vi "cno_check parameters.vi"(4 "initial parameters":dbl[](array[numeric]), 7 "tuning parameters":T7={"constraint weight"=1.0, "maximum minor iterations"=10}, 8 "error in (no error)":errorcluster, 9 "user defined functions":T2, 10 "limits":T5, 11 "state values":T6) -> (0 "error out":errorcluster, 1 "OB0":dbl[](array[numeric]), 2 "limits out":T5, 3 "state values out":T6, 5 "cno data":T1)   [LabVIEW 2017, in "NI_Gmath.lvlib"]
uses:
  <vilib>/gmath/NI_Gmath.lvlib
  <vilib>/gmath/NumericalOptimization/cno_initial values.ctl
  <vilib>/gmath/NumericalOptimization/cno_bounds.ctl
  <vilib>/gmath/NumericalOptimization/cno_tuning parameters.ctl
  <vilib>/gmath/NumericalOptimization/cno_user defined functions.ctl
  <vilib>/gmath/NumericalOptimization/cno_user objective function ref.ctl
  <vilib>/gmath/NumericalOptimization/objective function data.ctl
  <vilib>/gmath/NumericalOptimization/cno_data.ctl
  <vilib>/Analysis/7linalg.llb/Create Special Real Matrix.vi
  <vilib>/gmath/NumericalOptimization/zeroes_1d.vi
  <vilib>/Analysis/NI_AALPro.lvlib
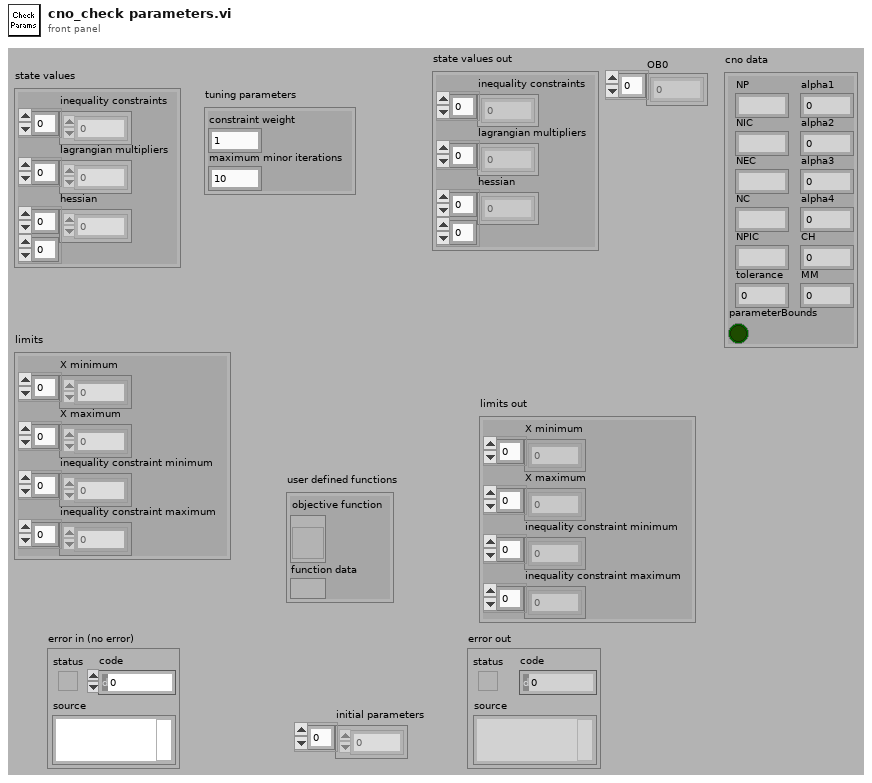
[diagram p1: front panel]
types:
  T1 = typedef "NI_Gmath.lvlib/cno_data.ctl" = cluster{"NP":i32, "NIC":i32, "NEC":i32, "NC":i32, "NPIC":i32, "parameterBounds":bool, "alpha1":dbl, "alpha2":dbl, "alpha3":dbl, "alpha4":dbl, "CH":i32, "MM":i32, "tolerance":dbl}
  T2 = typedef "NI_Gmath.lvlib/cno_user defined functions.ctl" = cluster{"objective function":T3, "function data":T4}
  T3 = typedef "NI_Gmath.lvlib/cno_user objective function ref.ctl" = refnum<vi>
  T4 = typedef "NI_Gmath.lvlib/objective function data.ctl" = variant
  T5 = typedef "NI_Gmath.lvlib/cno_bounds.ctl" = cluster{"X minimum":dbl[], "X maximum":dbl[], "inequality constraint minimum":dbl[], "inequality constraint maximum":dbl[]}
  T6 = typedef "NI_Gmath.lvlib/cno_initial values.ctl" = cluster{"inequality constraints":dbl[], "lagrangian multipliers":dbl[], "hessian":dbl[][]}
  T7 = typedef "NI_Gmath.lvlib/cno_tuning parameters.ctl" = cluster{"constraint weight":dbl, "maximum minor iterations":i32}
  T8 = enum32{"Identity", "Diagonal", "Toepliz", "Vandermonde", "Companion"}
  T9 = typedef "NI_Matrix.lvlib/RealMatrix.ctl" = dbl[][]
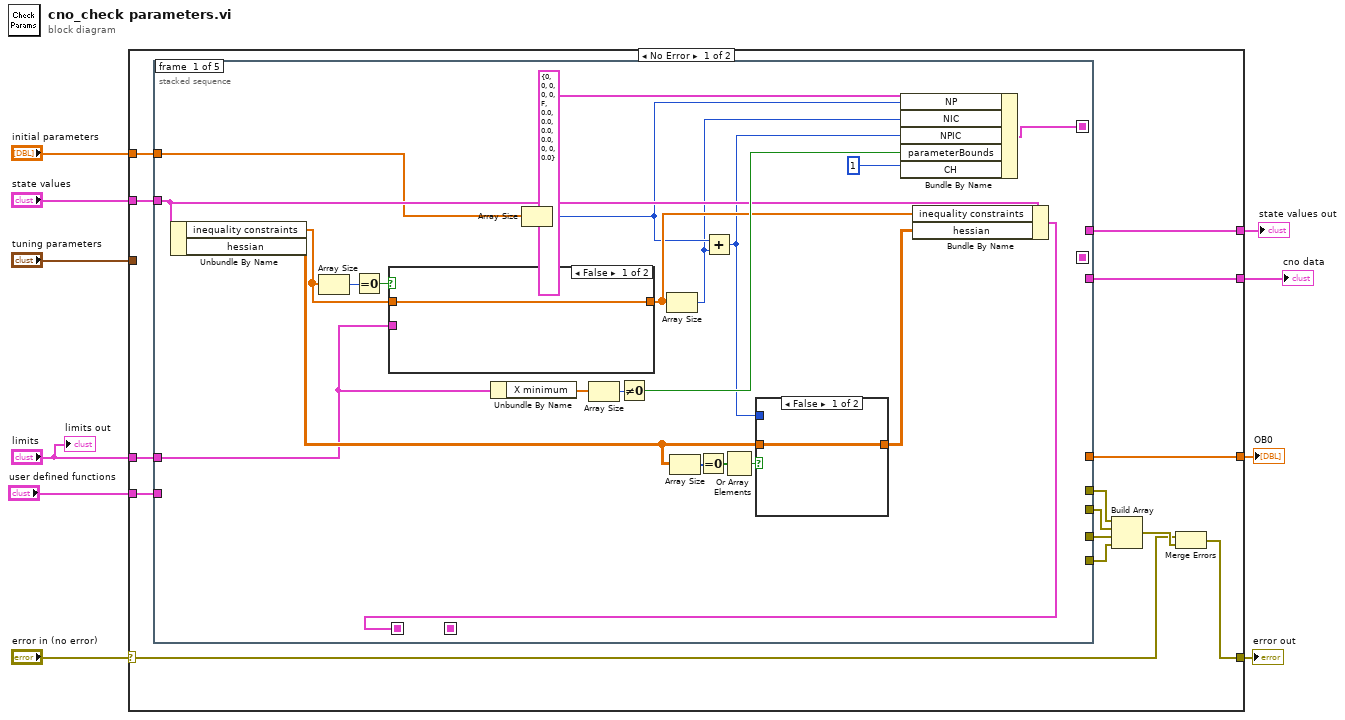
[diagram p0: block diagram]
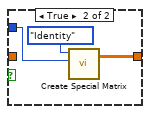
[diagram p2: hidden frame]
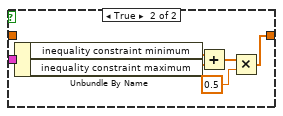
[diagram p3: hidden frame]
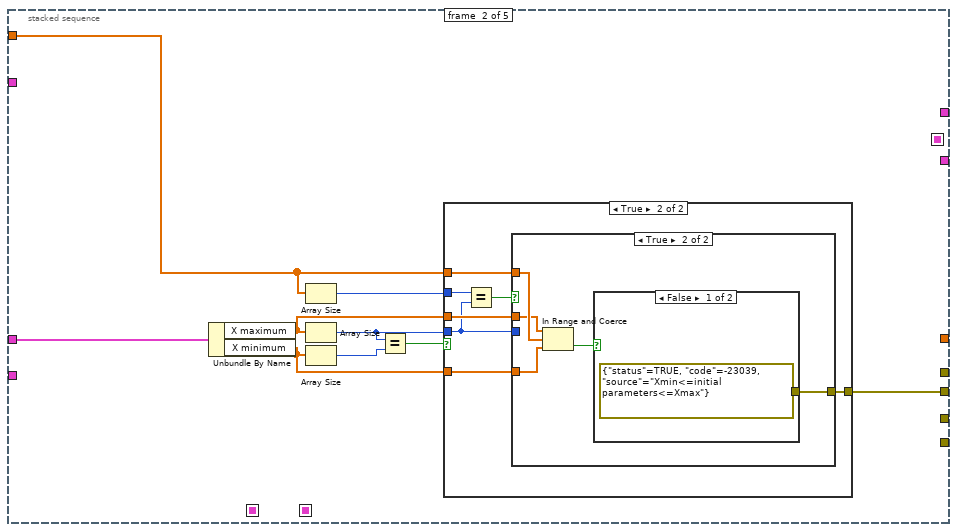
[diagram p4: hidden frame]
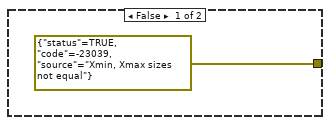
[diagram p5: hidden frame]
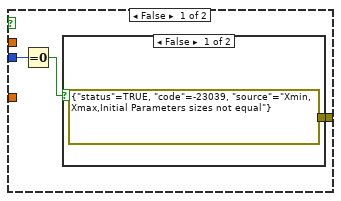
[diagram p6: hidden frame]
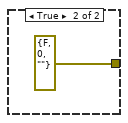
[diagram p8: hidden frame]
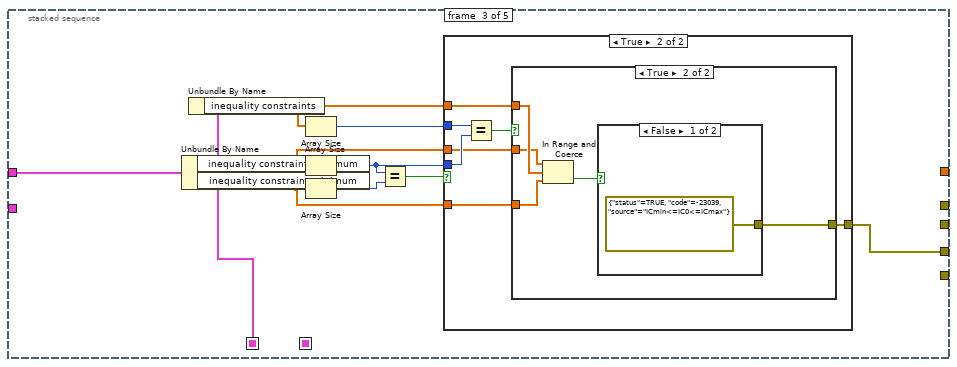
[diagram p9: hidden frame]
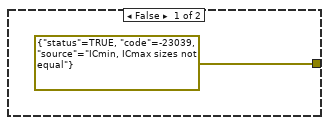
[diagram p10: hidden frame]
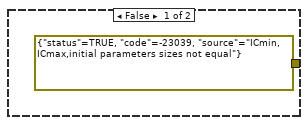
[diagram p11: hidden frame]
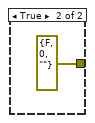
[diagram p12: hidden frame]
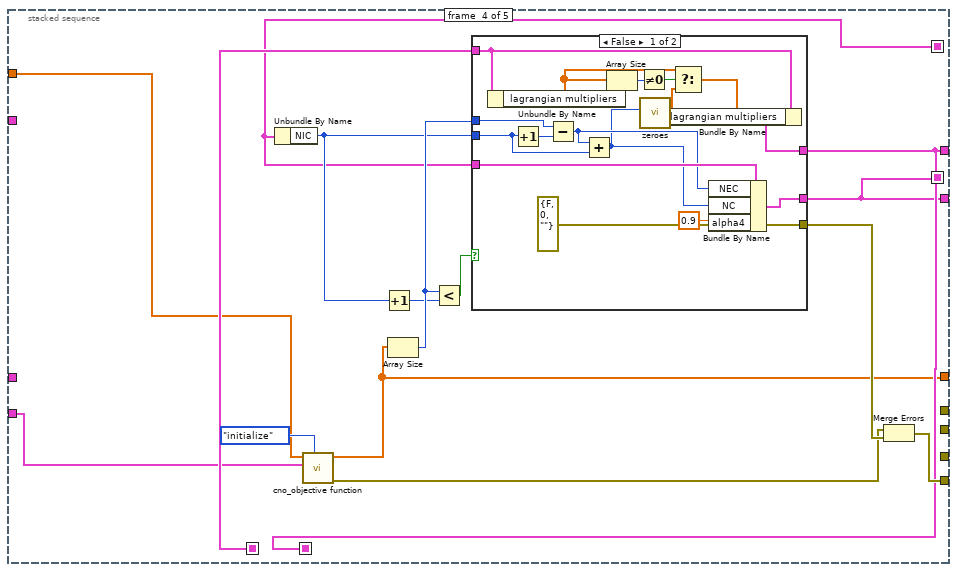
[diagram p13: hidden frame]
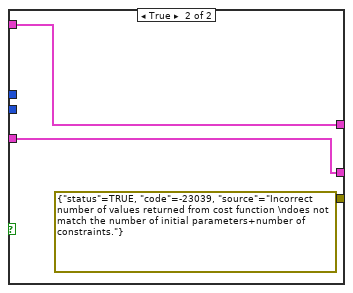
[diagram p14: hidden frame]
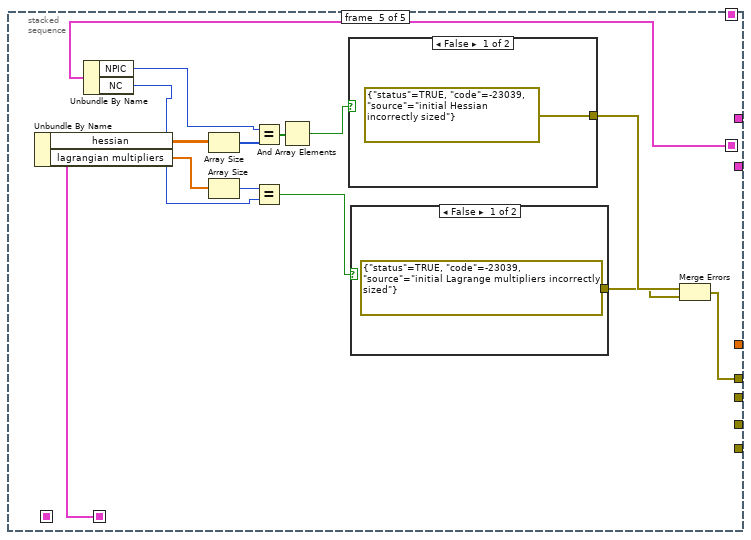
[diagram p15: hidden frame]
diagram:
  n1 = case shown="No Error" "error in (no error)" {
    selector: "error in (no error)" -> [w14 w162]
    tunnel: "tuning parameters" -> [_ _]
    tunnel: "state values" -> [w24 w163]
    tunnel: "limits" -> [w23 _]
    tunnel: [w22 w163] -> w7
    tunnel: [w21 w162] -> w6
    tunnel: [w20 _] -> w4
    tunnel: "user defined functions" -> [w19 _]
    tunnel: [w12 _] -> w2
    tunnel: "initial parameters" -> [w11 _]
    frame No Error {
      n2 = stacked-sequence {
        seq-local: [w40 _ _ _ _] -> [_ _ w86 w123 _]
        seq-local: [_ _ _ w121 _] -> [_ _ _ _ w159]
        seq-local: [w25 _ _ _ _] -> [_ _ _ w113 _]
        seq-local: [_ _ _ w112 _] -> [_ _ _ _ w146]
        tunnel: w24 -> [w45 _ _ _ _]
        tunnel: w23 -> [w31 w66 w95 _ _]
        tunnel: [_ _ _ w121 _] -> w22
        tunnel: [_ w60 _ _ _] -> w18
        tunnel: [_ _ w87 _ _] -> w17
        tunnel: [_ _ _ w115 _] -> w20
        tunnel: w19 -> [_ _ _ w114 _]
        tunnel: [_ _ _ w122 _] -> w16
        tunnel: [_ _ _ _ w149] -> w13
        tunnel: [_ _ _ w112 _] -> w12
        tunnel: w11 -> [w27 w58 _ w116 _]
        frame #0 {
          n3 = Unbundle By Name(w45) -> ("inequality constraints"=w42:dbl[], "hessian"=w35:dbl[][])
          n4 = Array Size(array=w42) -> (size(s)=w44:i32)
          n5 = Equal To 0?(x=w44) -> (x = 0?=w43:bool)
          n6 = case shown="False" w43 {
            tunnel: w31 -> [_ w57]
            tunnel: [w51 w52] -> w41
            tunnel: w42 -> [w51 _]
            frame False {
            }
            frame True {
              n7 = Unbundle By Name(w57) -> ("inequality constraint minimum"=w56:dbl[], "inequality constraint maximum"=w55:dbl[])
              n8 = Add(x=w56, y=w55) -> (x+y=w54:dbl[])
              n9 = Multiply(x=w54, y=0.5) -> (x*y=w52:dbl[])
            }
          }
          n10 = Unbundle By Name(w31) -> ("X minimum"=w30:dbl[])
          n11 = Array Size(array=w27) -> (size(s)=w34:i32)
          n12 = Array Size(array=w30) -> (size(s)=w29:i32)
          n13 = Not Equal To 0?(x=w29) -> (x != 0?=w46:bool)
          n14 = Array Size(array=w41) -> (size(s)=w33:i32)
          n15 = Array Size(array=w35) -> (size(s)=w39:i32[])
          n16 = Equal To 0?(x=w39) -> (x = 0?=w38:bool[])
          n17 = Add(x=w34, y=w33) -> (x+y=w32:i32)
          n18 = Or Array Elements(Boolean array=w38) -> (logical OR=w37:bool)
          n19 = case shown="False" w37 {
            tunnel: [w47 w49] -> w36
            tunnel: w35 -> [w47 _]
            tunnel: w32 -> [_ w48]
            frame False {
            }
            frame True {
              n20 = call-poly <vilib>:"Create Special Matrix.vi"("matrix type"=T8."Identity", "matrix size"=w48) -> ("Special Matrix"=w49:T9)  [unwired: 3 in, 1 out]
            }
          }
          n21 = Bundle By Name(cluster=T1 {"NP"=0, "NIC"=0, "NEC"=0, "NC"=0, "NPIC"=0, "parameterBounds"=FALSE, "alpha1"=0.0, "alpha2"=0.0, "alpha3"=0.0, "alpha4"=0.0, "CH"=0, "MM"=0, "tolerance"=0.0} ("cno data"), "NP"=w34, "NIC"=w33, "NPIC"=w32, "parameterBounds"=w46, "CH"=1) -> (w25:T1)
          n22 = Bundle By Name(cluster=w45, "inequality constraints"=w41, "hessian"=w36) -> (w40:T6)
        }
        frame #1 {
          n23 = Unbundle By Name(w66) -> ("X maximum"=w62:dbl[], "X minimum"=w61:dbl[])
          n24 = Array Size(array=w58) -> (size(s)=w63:i32)
          n25 = Array Size(array=w62) -> (size(s)=w59:i32)
          n26 = Array Size(array=w61) -> (size(s)=w65:i32)
          n27 = Equal?(x=w59, y=w65) -> (x = y?=w64:bool)
          n28 = case shown="True" w64 {
            tunnel: w63 -> [_ w74]
            tunnel: [errorcluster {"status"=TRUE, "code"=-23039, "source"="Xmin, Xmax sizes not equal"} ("error in (no error)") w72] -> w60
            tunnel: w59 -> [_ w68]
            tunnel: w62 -> [_ w71]
            tunnel: w61 -> [_ w70]
            tunnel: w58 -> [_ w69]
            frame False {
            }
            frame True {
              n29 = Equal?(x=w74, y=w68) -> (x = y?=w73:bool)
              n30 = case shown="True" w73 {
                tunnel: [w77 w79] -> w72
                tunnel: w71 -> [_ w81]
                tunnel: w70 -> [_ w82]
                tunnel: w69 -> [_ w83]
                tunnel: w68 -> [w76 _]
                frame False {
                  n31 = Equal To 0?(x=w76) -> (x = 0?=w75:bool)
                  n32 = case shown="False" w75 {
                    tunnel: [errorcluster {"status"=TRUE, "code"=-23039, "source"="Xmin, Xmax,Initial Parameters sizes not equal"} ("error in (no error)") _] -> w77
                    frame False {
                    }
                    frame True {
                    }
                  }
                }
                frame True {
                  n33 = In Range and Coerce(upper limit=w81, x=w83, lower limit=w82) -> (In Range?=w80:bool)  [unwired: 1 out]
                  n34 = case shown="False" w80 {
                    tunnel: [errorcluster {"status"=TRUE, "code"=-23039, "source"="Xmin<=initial parameters<=Xmax"} ("error in (no error)") errorcluster {"status"=FALSE, "code"=0, "source"=""} ("error in (no error)")] -> w79
                    frame False {
                    }
                    frame True {
                    }
                  }
                }
              }
            }
          }
        }
        frame #2 {
          n35 = Unbundle By Name(w95) -> ("inequality constraint maximum"=w90:dbl[], "inequality constraint minimum"=w89:dbl[])
          n36 = Unbundle By Name(w86) -> ("inequality constraints"=w88:dbl[])
          n37 = Array Size(array=w88) -> (size(s)=w92:i32)
          n38 = Array Size(array=w90) -> (size(s)=w91:i32)
          n39 = Array Size(array=w89) -> (size(s)=w94:i32)
          n40 = Equal?(x=w91, y=w94) -> (x = y?=w93:bool)
          n41 = case shown="True" w93 {
            tunnel: w92 -> [_ w103]
            tunnel: [errorcluster {"status"=TRUE, "code"=-23039, "source"="ICmin, ICmax sizes not equal"} ("error in (no error)") w100] -> w87
            tunnel: w91 -> [_ w102]
            tunnel: w90 -> [_ w99]
            tunnel: w89 -> [_ w98]
            tunnel: w88 -> [_ w97]
            frame False {
            }
            frame True {
              n42 = Equal?(x=w103, y=w102) -> (x = y?=w101:bool)
              n43 = case shown="True" w101 {
                tunnel: [errorcluster {"status"=TRUE, "code"=-23039, "source"="ICmin, ICmax,initial parameters sizes not equal"} ("error in (no error)") w105] -> w100
                tunnel: w99 -> [_ w107]
                tunnel: w98 -> [_ w108]
                tunnel: w97 -> [_ w109]
                frame False {
                }
                frame True {
                  n44 = In Range and Coerce(upper limit=w107, x=w109, lower limit=w108) -> (In Range?=w106:bool)  [unwired: 1 out]
                  n45 = case shown="False" w106 {
                    tunnel: [errorcluster {"status"=TRUE, "code"=-23039, "source"="ICmin<=IC0<=ICmax"} ("error in (no error)") errorcluster {"status"=FALSE, "code"=0, "source"=""} ("error in (no error)")] -> w105
                    frame False {
                    }
                    frame True {
                    }
                  }
                }
              }
            }
          }
        }
        frame #3 {
          n46 = Unbundle By Name(w113) -> ("NIC"=w120:i32)
          n47 = call <vilib>:"cno_objective function.vi"("function"=enum16{"initialize", "execute"}."initialize", "user defined functions"=w114, "X"=w116) -> ("error out"=w117:errorcluster, "F(X)"=w115:dbl[])  [unwired: 6 in, 1 out]
          n48 = Increment(x=w120) -> (x+1=w125:i32)
          n49 = Array Size(array=w115) -> (size(s)=w126:i32)
          n50 = Less?(x=w126, y=w125) -> (x < y?=w124:bool)
          n51 = case shown="False" w124 {
            tunnel: [errorcluster {"status"=FALSE, "code"=0, "source"=""} ("error out") errorcluster {"status"=TRUE, "code"=-23039, "source"="Incorrect number of values returned from cost function \ndoes not match the number of initial parameters+number of constraints."} ("error out")] -> w119
            tunnel: w123 -> [w138 w144]
            tunnel: w126 -> [w140 _]
            tunnel: w120 -> [w139 _]
            tunnel: [w132 w144] -> w121
            tunnel: w113 -> [w131 w143]
            tunnel: [w128 w143] -> w112
            frame False {
              n52 = Unbundle By Name(w138) -> ("lagrangian multipliers"=w135:dbl[])
              n53 = Increment(x=w139) -> (x+1=w141:i32)
              n54 = Subtract(x=w140, y=w141) -> (x-y=w130:i32)
              n55 = Add(x=w130, y=w139) -> (x+y=w129:i32)
              n56 = Array Size(array=w135) -> (size(s)=w137:i32)
              n57 = Not Equal To 0?(x=w137) -> (x != 0?=w136:bool)
              n58 = call-poly <vilib>:"zeroes.vi"("m"=w129) -> ("ones"=w134:dbl[])  [unwired: 7 in]
              n59 = Select(t=w135, s=w136, f=w134) -> (s? t:f=w133:dbl[])
              n60 = Bundle By Name(cluster=w138, "lagrangian multipliers"=w133) -> (w132:T6)
              n61 = Bundle By Name(cluster=w131, "NEC"=w130, "NC"=w129, "alpha4"=0.9) -> (w128:T1)
            }
            frame True {
            }
          }
          n62 = Merge Errors(w117, w119) -> (w122:errorcluster)
        }
        frame #4 {
          n63 = Unbundle By Name(w159) -> ("hessian"=w158:dbl[][], "lagrangian multipliers"=w157:dbl[])
          n64 = Unbundle By Name(w146) -> ("NPIC"=w148:i32, "NC"=w147:i32)
          n65 = Array Size(array=w158) -> (size(s)=w155:i32[])
          n66 = Array Size(array=w157) -> (size(s)=w156:i32)
          n67 = Equal?(x=w148, y=w155) -> (x = y?=w154:bool[])
          n68 = Equal?(x=w156, y=w147) -> (x = y?=w152:bool)
          n69 = And Array Elements(Boolean array=w154) -> (logical AND=w153:bool)
          n70 = case shown="False" w153 {
            tunnel: [errorcluster {"status"=TRUE, "code"=-23039, "source"="initial Hessian incorrectly sized"} ("error in (no error)") _] -> w151
            frame False {
            }
            frame True {
            }
          }
          n71 = case shown="False" w152 {
            tunnel: [errorcluster {"status"=TRUE, "code"=-23039, "source"="initial Lagrange multipliers incorrectly sized"} ("error in (no error)") _] -> w150
            frame False {
            }
            frame True {
            }
          }
          n72 = Merge Errors(w151, w150) -> (w149:errorcluster)
        }
      }
      n73 = Build Array(w13, w18, w17, w16) -> (w15:errorcluster[])
      n74 = Merge Errors(w14, w15) -> (w21:errorcluster)
    }
    frame Error {
    }
  }
  "error out" <- w6
  "state values out" <- w7
  "OB0" <- w4
  "cno data" <- w2
  "limits out" <- "limits"
